vi "aplikacja_projekt.vi"() -> ()   [LabVIEW 2022 SP3]
uses:
  <vilib>/Instr/_visa.llb/VISA Configure Serial Port (Instr).vi
  <vilib>/Utility/file.llb/Write Delimited Spreadsheet (string).vi
  <vilib>/Utility/file.llb/Read Delimited Spreadsheet (string).vi
panel:
  in  "Reset logi":bool
  in  "Odblokuj":bool
  in  "Zablokuj":bool
  out "Error zamkniecia/error out":errorcluster
  out "Ostatnie logi":string
  in  "Zmien haslo":bool
  out "Blad read/timeout osiagniety":errorcluster
  in  "Stop":bool
  in  "Nowy kod (4 liczby)":string
  in  "Wybierz Port":refnum<visa-resource-name>
  # "KONTROLA"
  # "LOGI"
  # "DEBUG"
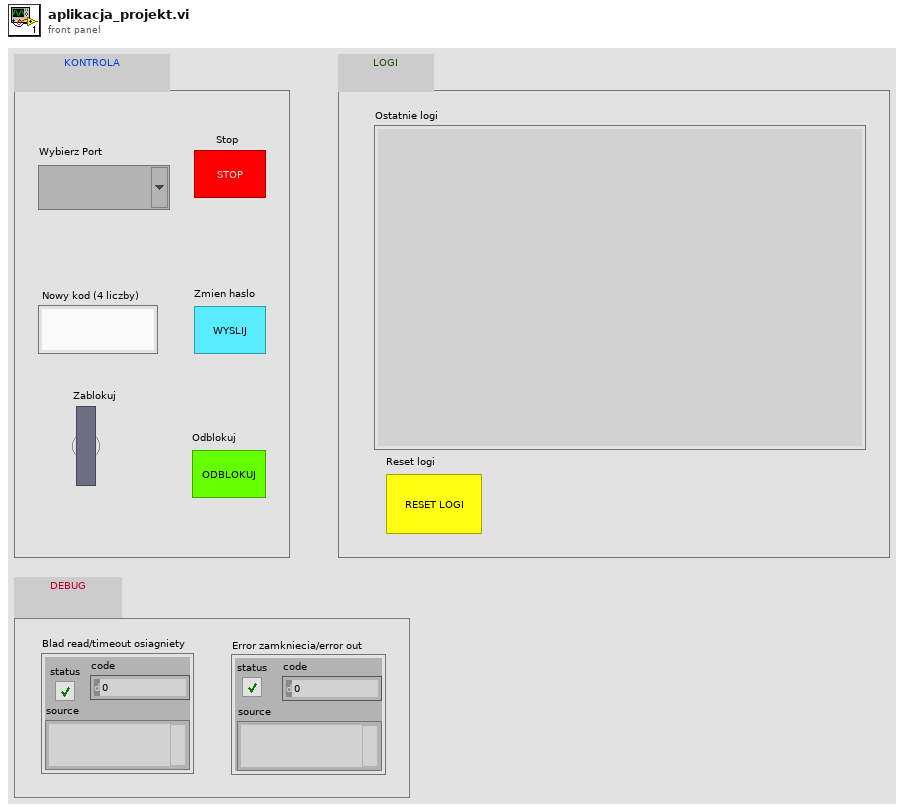
[diagram p1: front panel]
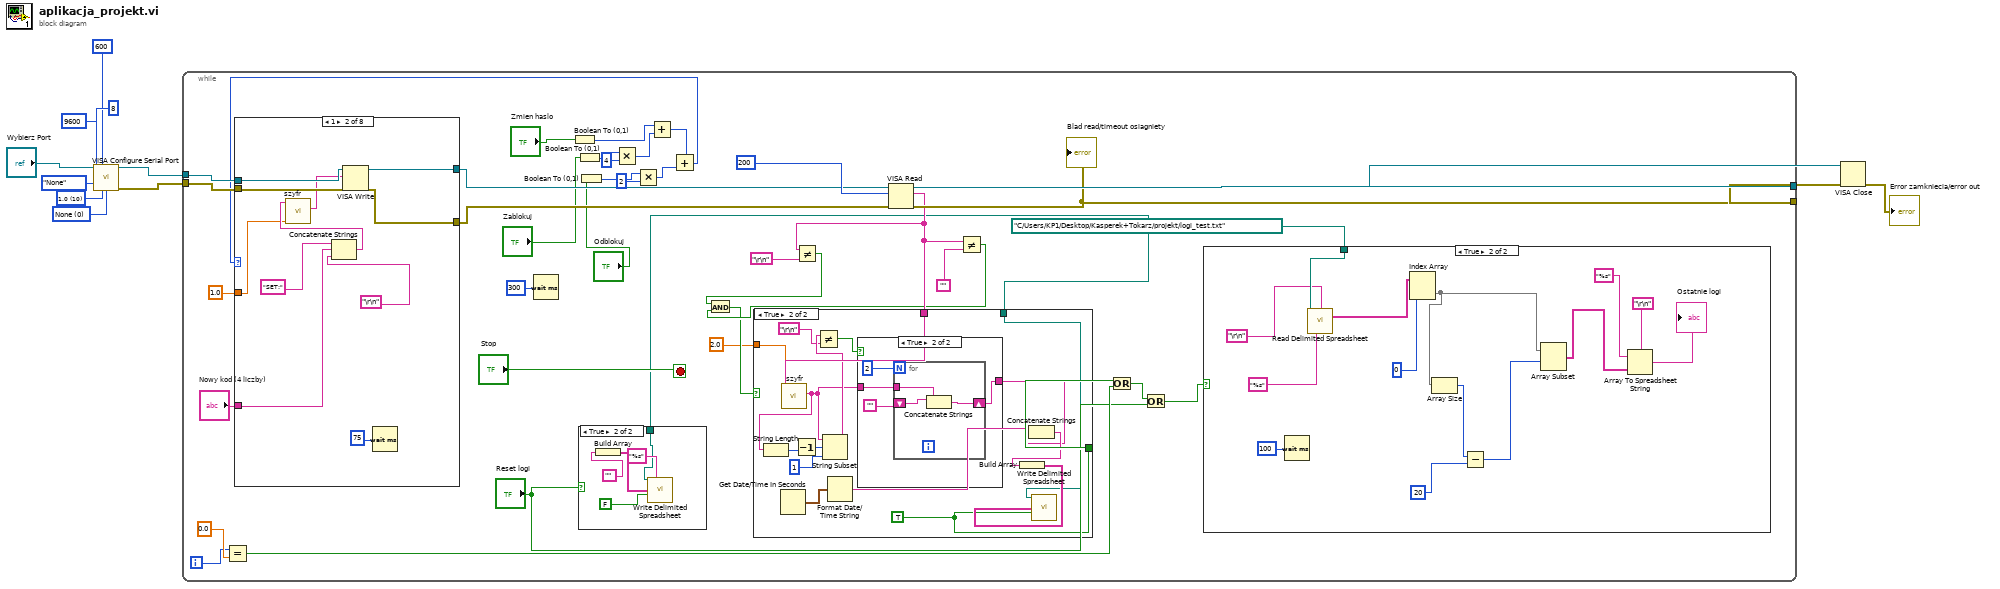
[diagram p0: block diagram]
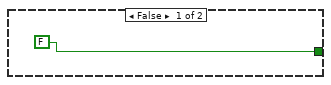
[diagram p4: hidden frame]
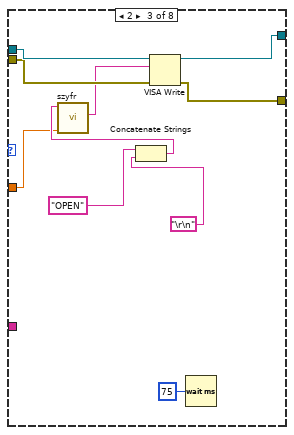
[diagram p7: hidden frame]
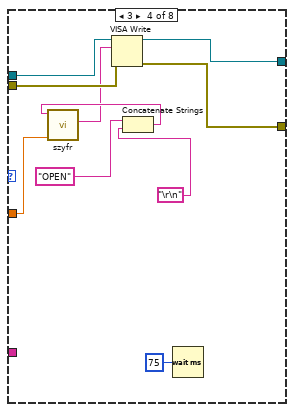
[diagram p8: hidden frame]
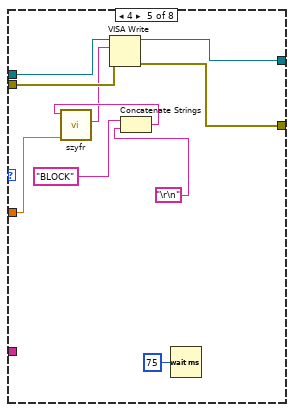
[diagram p9: hidden frame]
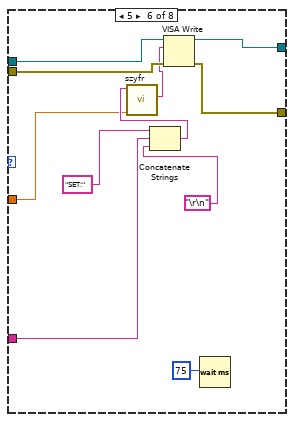
[diagram p10: hidden frame]
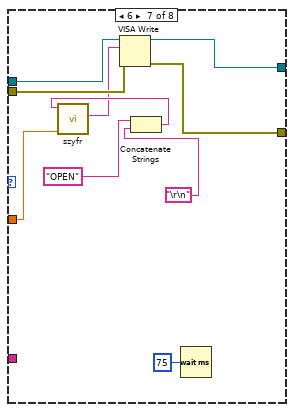
[diagram p11: hidden frame]
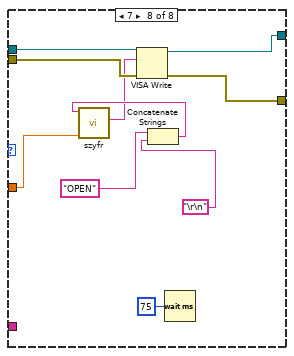
[diagram p12: hidden frame]
diagram:
  w3 = u16 0 items=["None", "XON/XOFF", "RTS/CTS", "XON/XOFF & RTS/CTS", "DTR/DSR", "XON/XOFF & DTR/DSR"] ("flow control (0:none)")
  w8 = u16 10 items=["1.0"=10, "1.5"=15, "2.0"=20] ("stop bits (10: 1 bit)")
  n1 = call-poly "VISA Configure Serial Port"("VISA resource name"="Wybierz Port", "timeout (10sec)"=u32 600, "baud rate (9600)"=u32 9600, "data bits (8)"=u16 8, "parity (0:none)"=enum16{"None", "Odd", "Even", "Mark", "Space"}."None", "stop bits (10: 1 bit)"=w8, "flow control (0:none)"=w3) -> ("VISA resource name out"=w7:refnum<visa-resource-name>, "error out"=w6:errorcluster)  [unwired: 7 in]
  n2 = while {
    tunnel: w7 -> [w50]
    tunnel: w6 -> [w49]
    tunnel: [w48] -> w5
    tunnel: [w47] -> w4
    i -> [w34]
    stop <- "Stop" stop-if-true
    w16 = path "C:/Users/KP1/Desktop/Kasperek+Tokarz/projekt/logi_test.txt" ("file path (dialog if empty)")
    n3 = Equal?(x=w34, y=0.0) -> (x = y?=w33:bool)
    n4 = Wait (ms)(milliseconds to wait=u32 300) -> ()  [unwired: 1 out]
    n5 = Boolean To (0,1)(Boolean="Zmien haslo") -> (0, 1=w24:i16)
    n6 = Boolean To (0,1)(Boolean="Zablokuj") -> (0, 1=w26:i16)
    n7 = Boolean To (0,1)(Boolean="Odblokuj") -> (0, 1=w22:i16)
    n8 = case shown="True" "Reset logi" {
      tunnel: w16 -> [_ w51]
      frame False {
      }
      frame True {
        n9 = Build Array("") -> (w52:string[])
        n10 = call-poly <vilib>:"Write Delimited Spreadsheet.vi"("file path (dialog if empty)"=w51, "format (%s)"="%s" ("format (%.3f)"), "1D data"=w52, "append to file? (new file:F)"=FALSE) -> ()  [unwired: 10 in, 2 out]
      }
    }
    n11 = Multiply(x=w26, y=i16 4) -> (x*y=w23:i16)
    n12 = Multiply(x=w22, y=i16 2) -> (x*y=w20:i16)
    n13 = Add(x=w24, y=w23) -> (x+y=w28:i16)
    n14 = Add(x=w28, y=w20) -> (x+y=w27:i16)
    n15 = case shown="1" w27 {
      tunnel: w50 -> [w96 w107 w114 w124 w134 w145 w155 w166]
      tunnel: w49 -> [w95 w106 w113 w123 w133 w144 w154 w165]
      tunnel: [w96 w105 w112 w122 w132 w143 w153 w164] -> w44
      tunnel: [w95 w104 w111 w121 w131 w142 w152 w163] -> w43
      tunnel: 1.0 ("Numeric") -> [_ w98 w109 w119 w129 w140 w150 w160]
      tunnel: "Nowy kod (4 liczby)" -> [_ w97 _ _ _ w138 _ _]
      frame 0, Default {
      }
      frame 1 {
        n16 = Concatenate Strings("SET:", w97, "\r\n") -> (w100:string)
        n17 = call "szyfr.vi"("Numeric"=w98, "String"=w100) -> ("String 2"=w99:string)  [unwired: 9 in]
        n18 = VISA Write(VISA resource name=w107, write buffer=w99, error in (no error)=w106) -> (VISA resource name out=w105:refnum<visa-resource-name>, error out=w104:errorcluster)  [unwired: 1 out]
        n19 = Wait (ms)(milliseconds to wait=u32 75) -> ()  [unwired: 1 out]
      }
      frame 2 {
        n20 = Concatenate Strings("OPEN", "\r\n") -> (w110:string)
        n21 = call "szyfr.vi"("Numeric"=w109, "String"=w110) -> ("String 2"=w108:string)  [unwired: 9 in]
        n22 = VISA Write(VISA resource name=w114, write buffer=w108, error in (no error)=w113) -> (VISA resource name out=w112:refnum<visa-resource-name>, error out=w111:errorcluster)  [unwired: 1 out]
        n23 = Wait (ms)(milliseconds to wait=u32 75) -> ()  [unwired: 1 out]
      }
      frame 3 {
        n24 = Concatenate Strings("OPEN", "\r\n") -> (w120:string)
        n25 = call "szyfr.vi"("Numeric"=w119, "String"=w120) -> ("String 2"=w118:string)  [unwired: 9 in]
        n26 = VISA Write(VISA resource name=w124, write buffer=w118, error in (no error)=w123) -> (VISA resource name out=w122:refnum<visa-resource-name>, error out=w121:errorcluster)  [unwired: 1 out]
        n27 = Wait (ms)(milliseconds to wait=u32 75) -> ()  [unwired: 1 out]
      }
      frame 4 {
        n28 = Concatenate Strings("BLOCK", "\r\n") -> (w130:string)
        n29 = call "szyfr.vi"("Numeric"=w129, "String"=w130) -> ("String 2"=w128:string)  [unwired: 9 in]
        n30 = VISA Write(VISA resource name=w134, write buffer=w128, error in (no error)=w133) -> (VISA resource name out=w132:refnum<visa-resource-name>, error out=w131:errorcluster)  [unwired: 1 out]
        n31 = Wait (ms)(milliseconds to wait=u32 75) -> ()  [unwired: 1 out]
      }
      frame 5 {
        n32 = Concatenate Strings("SET:", w138, "\r\n") -> (w141:string)
        n33 = call "szyfr.vi"("Numeric"=w140, "String"=w141) -> ("String 2"=w139:string)  [unwired: 9 in]
        n34 = VISA Write(VISA resource name=w145, write buffer=w139, error in (no error)=w144) -> (VISA resource name out=w143:refnum<visa-resource-name>, error out=w142:errorcluster)  [unwired: 1 out]
        n35 = Wait (ms)(milliseconds to wait=u32 75) -> ()  [unwired: 1 out]
      }
      frame 6 {
        n36 = Concatenate Strings("OPEN", "\r\n") -> (w151:string)
        n37 = call "szyfr.vi"("Numeric"=w150, "String"=w151) -> ("String 2"=w149:string)  [unwired: 9 in]
        n38 = VISA Write(VISA resource name=w155, write buffer=w149, error in (no error)=w154) -> (VISA resource name out=w153:refnum<visa-resource-name>, error out=w152:errorcluster)  [unwired: 1 out]
        n39 = Wait (ms)(milliseconds to wait=u32 75) -> ()  [unwired: 1 out]
      }
      frame 7 {
        n40 = Concatenate Strings("OPEN", "\r\n") -> (w161:string)
        n41 = call "szyfr.vi"("Numeric"=w160, "String"=w161) -> ("String 2"=w159:string)  [unwired: 9 in]
        n42 = VISA Write(VISA resource name=w166, write buffer=w159, error in (no error)=w165) -> (VISA resource name out=w164:refnum<visa-resource-name>, error out=w163:errorcluster)  [unwired: 1 out]
        n43 = Wait (ms)(milliseconds to wait=u32 75) -> ()  [unwired: 1 out]
      }
    }
    n44 = VISA Read(VISA resource name=w44, byte count=u32 200, error in (no error)=w43) -> (VISA resource name out=w48:refnum<visa-resource-name>, read buffer=w40:string, error out=w47:errorcluster)  [unwired: 1 out]
    "Blad read/timeout osiagniety" <- w47
    n45 = Not Equal?(x=w40, y="\r\n") -> (x != y?=w38:bool)
    n46 = Not Equal?(x=w40, y="") -> (x != y?=w37:bool)
    n47 = And(x=w38, y=w37) -> (x .and. y?=w36:bool)
    n48 = case shown="True" w36 {
      tunnel: w40 -> [_ w80]
      tunnel: w16 -> [_ w82]
      tunnel: [FALSE w81] -> w32
      tunnel: 2.0 ("Numeric") -> [_ w79]
      frame False {
      }
      frame True {
        w81 = TRUE ("append to file? (new file:F)")
        n49 = Get Date/Time In Seconds() -> (seconds since 1Jan1904=w86:timestamp)
        n50 = call "szyfr.vi"("Numeric"=w79, "String"=w80) -> ("String 2"=w71:string)  [unwired: 9 in]
        n51 = String Length(string=w71) -> (length=w77:i32)
        n52 = Decrement(x=w77) -> (x-1=w76:i32)
        n53 = String Subset(string=w71, offset (0)=w76, length (rest)=1 ("length (rest)")) -> (substring=w75:string)
        n54 = Not Equal?(x=w75, y="\r\n") -> (x != y?=w73:bool)
        n55 = Format Date/Time String(seconds (now)=w86) -> (date/time string=w85:string)  [unwired: 2 in]
        n56 = case shown="True" w73 {
          tunnel: [w87 w88] -> w72
          tunnel: w71 -> [w87 w90]
          frame False {
          }
          frame True {
            n57 = for {
              N: 2 -> [_]
              tunnel: w90 -> [w94]
              shift-right: [w93] -> w88
              shift-left: "" -> [w92]
              n58 = Concatenate Strings(w92, w94) -> (w93:string)
            }
          }
        }
        n59 = Concatenate Strings(w85, w72) -> (w84:string)
        n60 = Build Array(w84) -> (w83:string[])
        n61 = call-poly <vilib>:"Write Delimited Spreadsheet.vi"("file path (dialog if empty)"=w82, "1D data"=w83, "append to file? (new file:F)"=w81) -> ()  [unwired: 11 in, 2 out]
      }
    }
    n62 = Or(x=w32, y=w33) -> (x .or. y?=w14:bool)
    n63 = Or(x=w14, y="Reset logi") -> (x .or. y?=w13:bool)
    n64 = case shown="True" w13 {
      tunnel: w16 -> [_ w69]
      frame False {
      }
      frame True {
        n65 = Wait (ms)(milliseconds to wait=u32 100) -> ()  [unwired: 1 out]
        n66 = call-poly <vilib>:"Read Delimited Spreadsheet.vi"("file path (dialog if empty)"=w69, "format (%s)"="%s", "delimiter (\\t)"="\r\n") -> ("all rows"=w62:string[][])  [unwired: 7 in, 5 out]
        n67 = Index Array(array=w62, index (col)=0 ("disabled index (col)")) -> (element=w61:string[])  [unwired: 1 in]
        n68 = Array Size(array=w61) -> (size(s)=w59:i32)
        n69 = Subtract(x=w59, y=20) -> (x-y=w58:i32)
        n70 = Array Subset(array=w61, index=w58) -> (w63:string[])  [unwired: 1 in]
        n71 = Array To Spreadsheet String(delimiter (Tab)="\r\n", array=w63, 3:"%s" ("format string")) -> (spreadsheet string=→"Ostatnie logi":string)
      }
    }
  }
  n72 = VISA Close(VISA resource name=w5, error in (no error)=w4) -> (error out=→"Error zamkniecia/error out":errorcluster)
